vi "Add App Ref if Non-Existant.vi"(8 "error in (no error)":errorcluster, 10 "App Instances":T1[](array[typedef]), 11 "App Ref":refnum<vi>) -> (0 "error out":errorcluster, 1 "App Instance":T1, 2 "App Instances out":T1[](array[typedef]), 3 "App Ref out":refnum<vi>)   [LabVIEW 2020, in "MacroAssert.lvlib"]
doc: "Attempts to find <B>App Ref</B> within <B>App Instances</B>, and adds it if it does not exist."
uses:
  MacroAssert.lvlib
  CTLs/App Instance.ctl
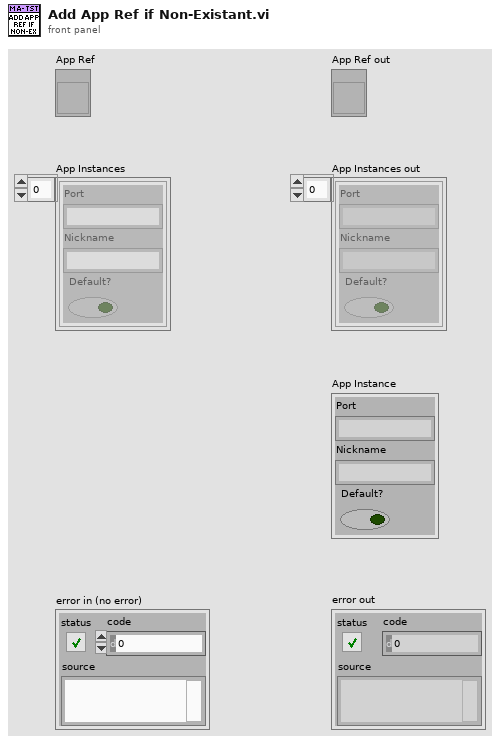
[diagram p1: front panel]
types:
  T1 = typedef "MacroAssert.lvlib/App Instance.ctl" = cluster{"Port":string, "Nickname":string, "Default?":bool}
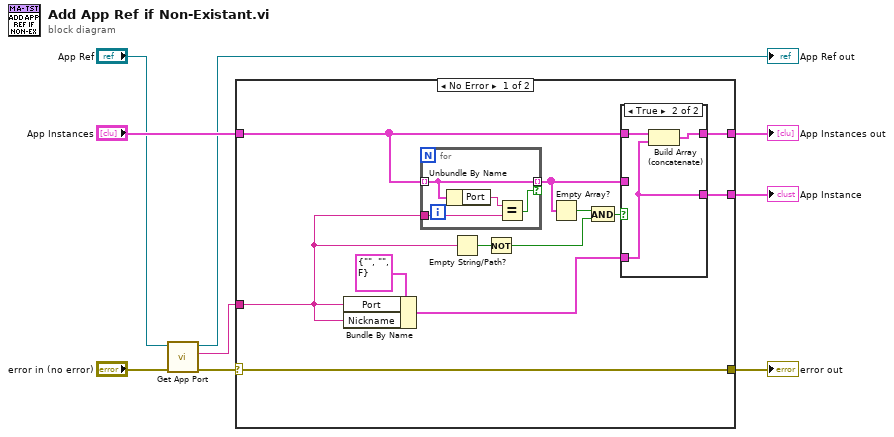
[diagram p0: block diagram]
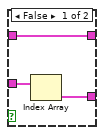
[diagram p2: hidden frame]
diagram:
  n1 = call "Get App Port.vi"("error in (no error)"="error in (no error)", "App Ref"="App Ref") -> ("error out"=w3:errorcluster, "Port"=w1:string, "App Ref out"=→"App Ref out":refnum<vi>)  [unwired: 7 in]
  n2 = case shown="No Error" w3 {
    selector: w3 -> [w10 w32]
    tunnel: "App Instances" -> [w15 w33]
    tunnel: [w13 w33] -> w8
    tunnel: [w12 _] -> w7
    tunnel: w1 -> [w11 _]
    tunnel: [w10 w32] -> w6
    frame No Error {
      n3 = Bundle By Name(cluster=T1 {"Port"="", "Nickname"="", "Default?"=FALSE} ("App Instance"), "Port"=w11, "Nickname"=w11) -> (w18:T1)
      n4 = for {
        tunnel: w15 -> [w29] mode=indexing
        tunnel: [w29] -> w14 mode=indexing if=w28
        tunnel: w11 -> [w30]
        n5 = Unbundle By Name(w29) -> ("Port"=w31:string)
        n6 = Equal?(x=w31, y=w30) -> (x = y?=w28:bool)
      }
      n7 = Empty String/Path?(string/path=w11) -> (empty?=w21:bool)
      n8 = Not(x=w21) -> (.not. x?=w20:bool)
      n9 = Empty Array?(array=w14) -> (empty?=w16:bool)
      n10 = And(x=w16, y=w20) -> (x .and. y?=w19:bool)
      n11 = case shown="True" w19 {
        tunnel: w15 -> [w24 w27]
        tunnel: [w24 w26] -> w13
        tunnel: w18 -> [_ w25]
        tunnel: w14 -> [w23 _]
        tunnel: [w22 w25] -> w12
        frame False {
          n12 = Index Array(array=w23) -> (element=w22:T1)  [unwired: 1 in]
        }
        frame True {
          n13 = Build Array (concatenate)(w27, w25) -> (w26:T1[])
        }
      }
    }
    frame Error {
    }
  }
  "App Instances out" <- w8
  "error out" <- w6
  "App Instance" <- w7
